vi "forget and finalize prepared statements.vi"(8 "error in (no error)":errorcluster, 10 "ppDb":i64, 11 "pStmt":i64) -> (0 "error out":errorcluster, 3 "error?":bool)   [LabVIEW 2014, in "SQLite3LV.lvlib" / "sqlite3.lvclass"]
uses:
  sqlite3.lvclass
  SQLite3LV.lvlib
  sqlite3_64.dll
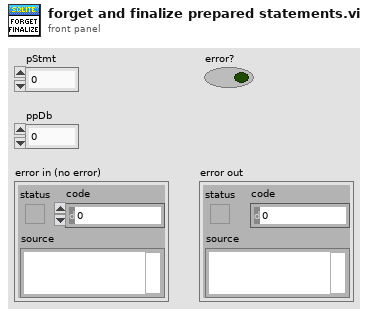
[diagram p1: front panel]
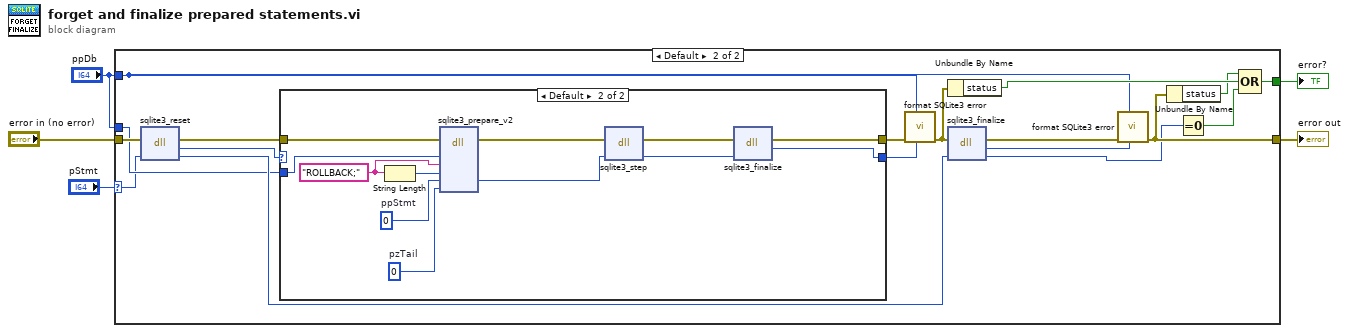
[diagram p0: block diagram]
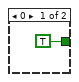
[diagram p2: hidden frame]
diagram:
  n1 = case shown="Default" "pStmt" {
    selector: "pStmt" -> [_ w8]
    tunnel: [TRUE w22] -> w1
    tunnel: [_ w20] -> w2
    tunnel: "error in (no error)" -> [_ w17]
    tunnel: "ppDb" -> [_ w15]
    tunnel: "ppDb" -> [_ w12]
    frame 0 {
    }
    frame Default {
      n2 = dll-call lib="C:/Users/BobUser/Desktop/LVTables/sqlite3**.*" fn="sqlite3_reset"(error in=w17, "pStmt"=w8) -> (error out=w9:errorcluster, "result code"=w13:i32, "pStmt"=w16:i64)  [unwired: 2 in, 1 out]
      n3 = case shown="Default" w13 {
        selector: w13 -> [w26 _]
        tunnel: w12 -> [_ w37]
        tunnel: [w25 w30] -> w11
        tunnel: [w26 w29] -> w10
        tunnel: w9 -> [w25 w28]
        frame 0 {
        }
        frame Default {
          w27 = i64 0  # pzTail
          w36 = "ROLLBACK;" ("zSql")
          w38 = i64 0  # ppStmt
          n4 = String Length(string=w36) -> (length=w35:i32)
          n5 = dll-call lib="C:/Users/BobUser/Desktop/LVTables/sqlite3**.*" fn="sqlite3_prepare_v2"(error in=w28, "pdb"=w37, "zSql"=w36, "nByte"=w35, "ppStmt"=w38, "pzTail"=w27) -> (error out=w31:errorcluster, "ppStmt"=w34:i64)  [unwired: 7 in, 1 out]
          n6 = dll-call lib="C:/Users/BobUser/Desktop/LVTables/sqlite3**.*" fn="sqlite3_step"(error in=w31, "pStmt"=w34) -> (error out=w32:errorcluster, "pStmt"=w33:i64)  [unwired: 3 in, 1 out]
          n7 = dll-call lib="C:/Users/BobUser/Desktop/LVTables/sqlite3**.*" fn="sqlite3_finalize"(error in=w32, "pStmt"=w33) -> (error out=w30:errorcluster, "result"=w29:i32)  [unwired: 3 in, 1 out]
        }
      }
      n8 = call "format SQLite3 error.vi"("SQLite3LV Connection result"=w10, "ppDb"=w15, "error in (no error)"=w11) -> ("error out"=w14:errorcluster)  [unwired: 8 in]
      n9 = Unbundle By Name(w14) -> ("status"=w24:bool)
      n10 = dll-call lib="C:/Users/BobUser/Desktop/LVTables/sqlite3**.*" fn="sqlite3_finalize"(error in=w14, "pStmt"=w16) -> (error out=w7:errorcluster, "result"=w21:i32, "pStmt"=w18:i64)  [unwired: 2 in, 1 out]
      n11 = call "format SQLite3 error.vi"("SQLite3LV Connection result"=w21, "ppDb"=w15, "error in (no error)"=w7) -> ("error out"=w20:errorcluster)  [unwired: 8 in]
      n12 = Unbundle By Name(w20) -> ("status"=w19:bool)
      n13 = Equal To 0?(x=w18) -> (x = 0?=w23:bool)
      n14 = Compound Arithmetic op=OR(w19, w24, w23) -> (w22:bool)
    }
  }
  "error out" <- w2
  "error?" <- w1
